vi "manual_wait.vi"(5 "change_in_event":refnum<user-event>, 7 "waitgroup":T1, 8 "error in (no error)":errorcluster, 11 "data":variant) -> (0 "error out":errorcluster)   [LabVIEW 2015, in "example_01.lvlib"]
uses:
  example_01.lvlib
  <userlib>/antonio-alexander/lv-waitgroup/public/_controls/api_waitgroup.ctl
  lv-recipe-machine/public/_controls/change.ctl
  _controls/steps_actions.ctl
  _controls/steps_actions_data.ctl
  lv-recipe-machine/lv-recipe-machine.lvlib
  <userlib>/antonio-alexander/lv-waitgroup/lv-waitgroup.lvlib
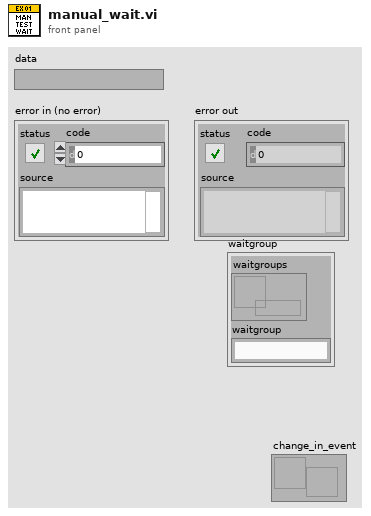
[diagram p1: front panel]
types:
  T1 = typedef "lv-waitgroup.lvlib/api_waitgroup.ctl" = cluster{"waitgroups":refnum<data-value>, "waitgroup":string}
  T2 = typedef "example_01.lvlib/steps_actions_data.ctl" = cluster{"step_action":T3, "data":variant}
  T3 = typedef "example_01.lvlib/steps_actions.ctl" = enum16{"<steps_actions>", "manual_random", "manual_comparison", "manual_wait", "auto_random", "auto_wait", "criteria_initialize", "criteria_count", "criteria_comparison", "transition_simple", "transition_count", "transition_comparison", "<null>"}
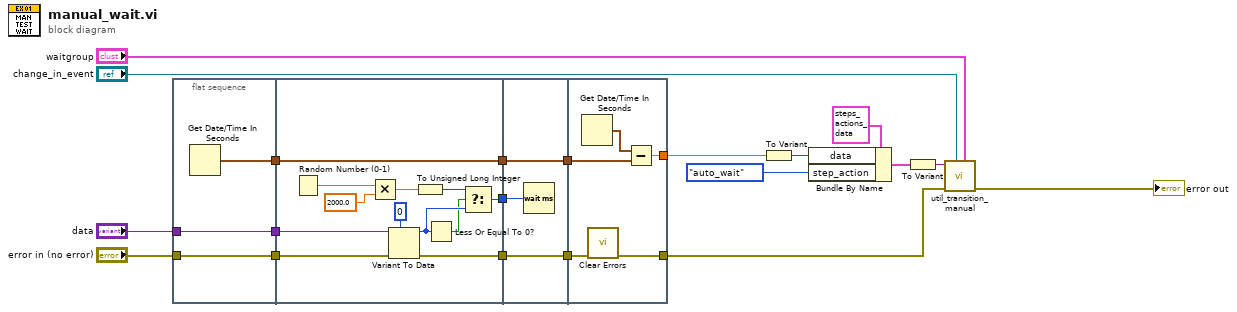
[diagram p0: block diagram]
diagram:
  n1 = flat-sequence {
    tunnel: "data" -> [w23]
    tunnel: "error in (no error)" -> [w22]
    tunnel: [w23] -> w17
    tunnel: [w22] -> w16
    tunnel: [w21] -> w15
    tunnel: w17 -> [w28]
    tunnel: w16 -> [w29]
    tunnel: w15 -> [w35]
    tunnel: [w35] -> w14
    tunnel: [w27] -> w12
    tunnel: [w24] -> w7
    tunnel: w14 -> [w38]
    tunnel: [w38] -> w13
    tunnel: w12 -> [w37]
    tunnel: [w36] -> w8
    tunnel: w7 -> [w36]
    tunnel: w13 -> [w42]
    tunnel: [w41] -> w11
    tunnel: [w40] -> w9
    tunnel: w8 -> [w39]
    frame #0 {
      n2 = Get Date/Time In Seconds() -> (seconds since 1Jan1904=w21:timestamp)
    }
    frame #1 {
      n3 = Random Number (0-1)() -> (number: 0 to 1=w31:dbl)
      n4 = Multiply(x=w31, y=2000.0) -> (x*y=w33:dbl)
      n5 = Variant To Data(error in=w29, type=u32 0, Variant=w28) -> (data=w26:u32, error out=w24:errorcluster)
      n6 = To Unsigned Long Integer(number=w33) -> (unsigned 32bit integer=w34:u32)
      n7 = Less Or Equal To 0?(x=w26) -> (x <= 0?=w25:bool)
      n8 = Select(t=w34, s=w25, f=w26) -> (s? t:f=w27:u32)
    }
    frame #2 {
      n9 = Wait (ms)(milliseconds to wait=w37) -> ()  [unwired: 1 out]
    }
    frame #3 {
      n10 = Get Date/Time In Seconds() -> (seconds since 1Jan1904=w43:timestamp)
      n11 = call <vilib>:"Clear Errors.vi"("error in (no error)"=w39) -> ("error out"=w40:errorcluster)  [unwired: 5 in, 1 out]
      n12 = Subtract(x=w43, y=w42) -> (x-y=w41:dbl)
    }
  }
  n13 = To Variant(anything=w11) -> (Variant=w20:variant)
  n14 = Bundle By Name(cluster=T2 {"step_action"=enum."<steps_actions>", "data"=variant} ("step_data"), "data"=w20, "step_action"=steps_actions."auto_wait" ("manual_action")) -> (w10:T2)
  n15 = To Variant(anything=w10) -> (Variant=w6:variant)
  n16 = call "util_transition_manual.vi"("api_waitgroup"="waitgroup", "change_in_event"="change_in_event", "error in (no error)"=w9, "data"=w6) -> ("error out"=→"error out":errorcluster)  [unwired: 7 in]
